vi "Configure Relay Polarity.vi"(8 "error in (no error)":errorcluster {"code" format="%.0x"}, 9 "Relay Polarity (0: Normal)":i32(ring) items=["Reverse"=1, "Normal"=0], 10 "Channel Name (1)":string="1", 11 "VISA resource name":refnum<visa-resource-name>) -> (0 "error out":errorcluster {"code" format="%.0x"}, 3 "VISA resource name out":refnum<visa-resource-name>)   [LabVIEW 2010, in "Agilent N6700 Series.lvlib"]
doc: "Sets the output relay polarity.\n\n<b>Note:</b>\n\nThe function is valid only when your instrument installs Option 760."
uses:
  Agilent N6700 Series.lvlib
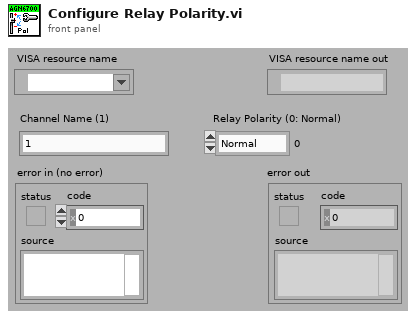
[diagram p1: front panel]
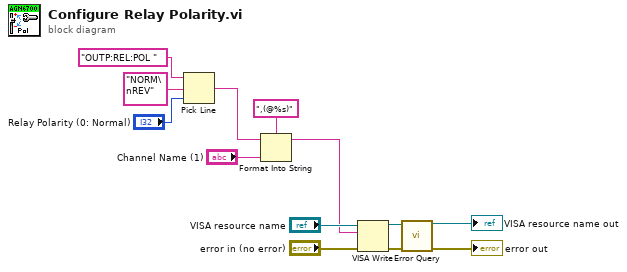
[diagram p0: block diagram]
diagram:
  n1 = Pick Line(string ("")="OUTP:REL:POL ", multi-line string="NORM\nREV", line index="Relay Polarity (0: Normal)") -> (output string=w10:string)
  n2 = Format Into String(format string=",(@%s)", initial string=w10, "Channel Name (1)") -> (resulting string=w5:string)  [unwired: 1 in, 1 out]
  n3 = VISA Write(VISA resource name="VISA resource name", write buffer=w5, error in (no error)="error in (no error)") -> (VISA resource name out=w4:refnum<visa-resource-name>, error out=w3:errorcluster)  [unwired: 1 out]
  n4 = call "Error Query.vi"("VISA resource name"=w4, "error in (no error)"=w3) -> ("VISA resource name out"=→"VISA resource name out":refnum<visa-resource-name>, "error out"=→"error out":errorcluster)  [unwired: 10 in, 2 out]
